vi "Recurse.vi"(8 "Error in":errorcluster, 10 "Msg DVR in":refnum<data-value>, 11 "TEMPLATE Actor in":refnum<class "{{Name}}Actor.lvclass">) -> (0 "Error out":errorcluster, 2 "Msg DVR out":refnum<data-value>, 3 "TEMPLATE Actor out":refnum<class "{{Name}}Actor.lvclass">)   [LabVIEW 2020, in "_Template.lvlib" / "Templates.lvlib" / "{{Name}}Actor.lvlib" / "{{Name}}Actor.lvclass"]
uses:
  {{Name}}Actor.lvclass
  {{Name}}Actor.lvclass/{{Name}}Actor.ctl
  jettl/jettl/Message/Message.lvclass
  jettl/jettl/Actor/Actor.lvclass
  jettl/jettl/jettl.lvlib
  jettl/jettl/Message.ctl
panel:
  # "This front panel should not be manipulated."
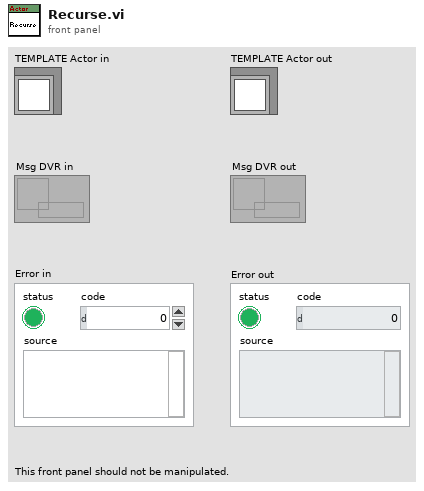
[diagram p1: front panel]
types:
  T1 = typedef "jettl.lvlib/Message.ctl" = cluster{"Message":refnum<class "Message.lvclass">}
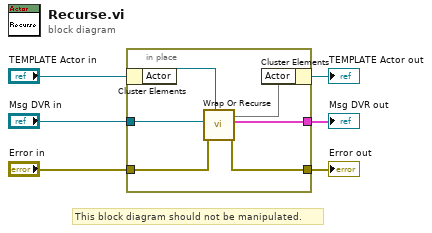
[diagram p0: block diagram]
diagram:
  # "This block diagram should not be manipulated."
  n1 = in-place {
    in-place-border: [w9] -> w6
    in-place-border: "Error in" -> [w10]
    in-place-border: "Msg DVR in" -> [w8]
    in-place-border: [w7] -> w1
    n2 = in-place-cluster #1("TEMPLATE Actor in") -> ("Actor"=w12:refnum<class "Actor.lvclass">)
    n3 = call "Wrap Or Recurse.vi"(7:w12, "Error in"=w10, "Message in"=w8) -> ("Error out"=w9:errorcluster, "Message out"=w7:T1, 5:w11)  [unwired: 5 in, 1 out]
    n4 = in-place-cluster #1("Actor"=w11) -> (→"TEMPLATE Actor out":refnum<class "{{Name}}Actor.lvclass">)
  }
  "Error out" <- w6
  "Msg DVR out" <- w1
